vi "Recover Config.vi"(8 "error in":errorcluster, 11 "Philips UI in":refnum<class "Flex UI.lvclass">) -> (0 "error out":errorcluster, 3 "Philips UI out":refnum<class "Flex UI.lvclass">)   [LabVIEW 2014, in "Flex UI.lvclass"]
uses:
  Flex UI.lvclass
  Flex UI.lvclass/Flex UI.ctl
  <userlib>/_OpenG.lib/file/file.llb/File Exists - Scalar__ogtk.vi
  <vilib>/Utility/config.llb/NI_LVConfig.lvlib
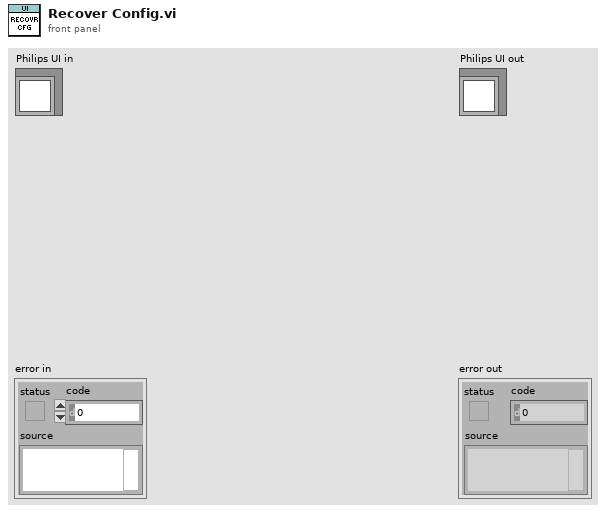
[diagram p1: front panel]
types:
  T1 = typedef "NI_LVConfig.lvlib/Config Data RefNum.ctl" = refnum<k1>
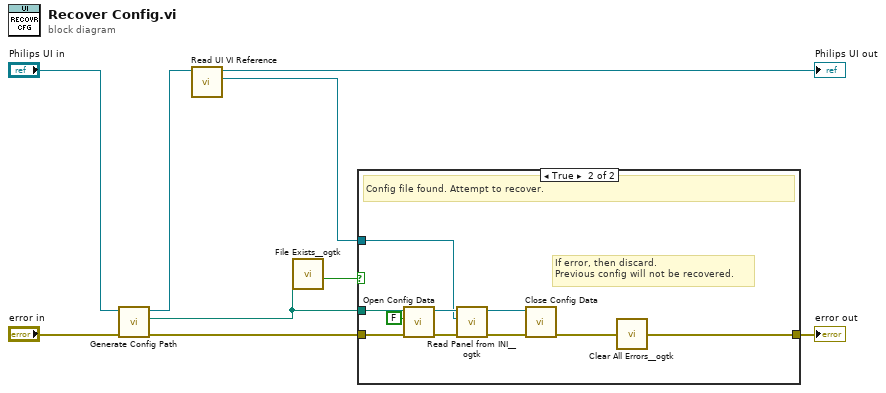
[diagram p0: block diagram]
diagram:
  n1 = call-dynamic "Generate Config Path.vi"("error in"="error in", "Philips UI in"="Philips UI in") -> ("error out"=w4:errorcluster, "Config Path"=w1:path, "Philips UI out"=w5:refnum<class "Flex UI.lvclass">)  [unwired: 7 in]
  n2 = call "Read UI VI Reference.vi"("Philips UI in"=w5) -> ("UI VI Reference"=w2:refnum<vi>, "Philips UI out"=→"Philips UI out":refnum<class "Flex UI.lvclass">)  [unwired: 9 in]
  n3 = call-poly <userlib>:"File Exists__ogtk.vi"("file path"=w1) -> ("exists"=w8:bool)  [unwired: 6 in, 1 out]
  n4 = case shown="True" w8 {
    tunnel: w2 -> [_ w16]
    tunnel: w4 -> [w10 w15]
    tunnel: [w10 w11] -> w6
    tunnel: w1 -> [_ w12]
    frame False {
      # "No config data. Do nothing."
    }
    frame True {
      # "If error, then discard.\nPrevious config will not be recovered."
      # "Config file found. Attempt to recover."
      n5 = call <vilib>:"Open Config Data.vi"("error in (no error)"=w15, "create file if necessary (T)"=FALSE, "configuration file path"=w12) -> ("error out"=w18:errorcluster, "refnum"=w17:T1)  [unwired: 6 in, 1 out]
      n6 = call <userlib>:"Read Panel from INI__ogtk.vi"("error in (no error)"=w18, "VI ref"=w16, "refnum"=w17) -> ("error out"=w19:errorcluster, "refnum out"=w20:T1)  [unwired: 7 in]
      n7 = call <vilib>:"Close Config Data.vi"("error in (no error)"=w19, "refnum"=w20) -> ("error out"=w14:errorcluster)  [unwired: 8 in, 1 out]
      n8 = call <userlib>:"Clear All Errors__ogtk.vi"("Error In"=w14) -> ("Error Out"=w11:errorcluster)  [unwired: 3 in]
    }
  }
  "error out" <- w6
